vi "Line fit.vi"() -> ()   [LabVIEW 2016]
uses:
  <vilib>/Analysis/NI_AALPro.lvlib
panel:
  out "Intercept":dbl
  out "Slope":dbl
  in  "Channels":string[](array[string])=["Bdot", "Btilt"]
  in  "File Path":path
  out "XY Graph":cluster{dbl[], dbl[]}[](graph)
  # "X\nY"
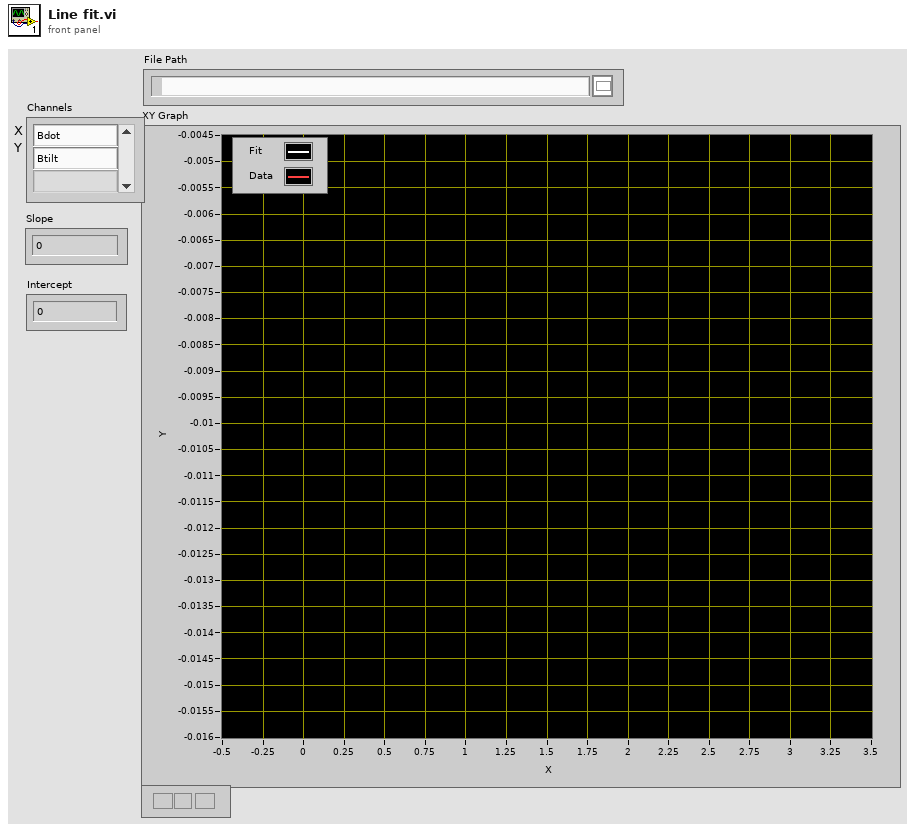
[diagram p1: front panel]
types:
  T1 = enum16{"open", "open or create", "create or replace", "create", "open (read-only)"}
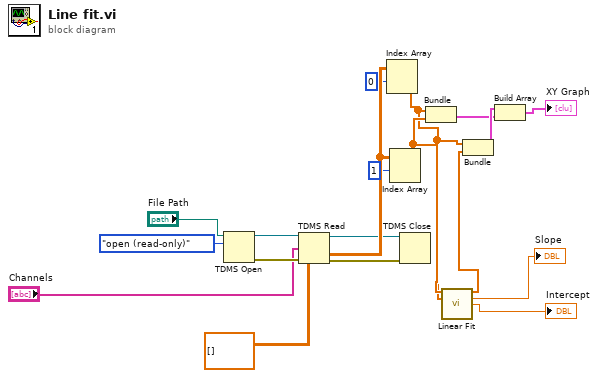
[diagram p0: block diagram]
diagram:
  n1 = TDMS Open(10:T1."open (read-only)" ("operation (0:open)"), 11:"File Path") -> (0:w16:errorcluster, 3:w17:refnum<k34>)  [unwired: 5 in]
  n2 = TDMS Read(0:w17, 7:"Channels", 11:w16, 12:dbl[][] []) -> (4:w9:refnum<k34>, 10:w13:dbl[][], 15:w10:errorcluster)  [unwired: 4 in, 3 out]
  n3 = Index Array(array=w13, index (row)=0) -> (element=w7:dbl[])  [unwired: 1 in]
  n4 = Index Array(array=w13, index (row)=1) -> (element=w8:dbl[])  [unwired: 1 in]
  n5 = TDMS Close(8:w10, 11:w9) -> ()  [unwired: 2 out]
  n6 = Bundle(w7, w8) -> (w4:cluster{dbl[], dbl[]})  [unwired: 1 in]
  n7 = call <vilib>:"Linear Fit.vi"("Y"=w8, "X"=w7) -> ("Best Linear Fit"=w6:dbl[], "slope"=→"Slope":dbl, "intercept"=→"Intercept":dbl)  [unwired: 9 in, 2 out]
  n8 = Bundle(w7, "Best Linear Fit"=w6) -> (w5:cluster{dbl[], "Best Linear Fit":dbl[]})  [unwired: 1 in]
  n9 = Build Array(w5, w4) -> (→"XY Graph":cluster{dbl[], "Best Linear Fit":dbl[]}[])
